vi "intersection_counter.vi"(8 "Booleanos e Contadores Iniciais":T1={"Correct"=FALSE, "Enable State change"=TRUE, "First End"=FALSE, "Intersections crossed"=0.0, "Intersections crossed total"=0.0, "Bonecos"=0.0} caption="Booleanos e Contadores") -> (2 "Intersections crossed":dbl)   [LabVIEW 2016]
uses:
  booleanos.ctl
panel:
  # "Permite que ocorra troca \nde estados se True e interrompe-as \nse False."
  # "Booleano que retorna F quando chega em Delivery.\nGarantindo que não contará\nmais intersections"
  # "Salva o total de interseções \ncruzadas"
  # "Contador de quantas \ninterseções foram cruzadas.\nSoma ao acertar"
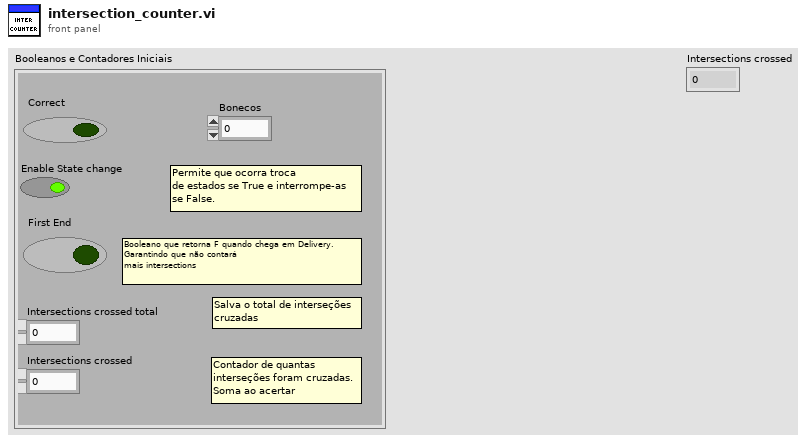
[diagram p1: front panel]
types:
  T1 = typedef "booleanos.ctl" = cluster{"Correct":bool, "Enable State change":bool, "First End":bool, "Intersections crossed":dbl, "Intersections crossed total":dbl, "Bonecos":dbl}
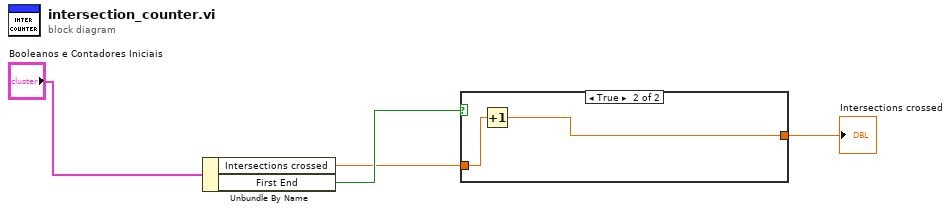
[diagram p0: block diagram]
diagram:
  n1 = Unbundle By Name("Booleanos e Contadores Iniciais") -> ("Intersections crossed"=w3:dbl, "First End"=w4:bool)
  n2 = case shown="True" w4 {
    tunnel: w3 -> [w5 w7]
    tunnel: [w5 w6] -> w2
    frame False {
    }
    frame True {
      n3 = Increment(x=w7) -> (x+1=w6:dbl)
    }
  }
  "Intersections crossed" <- w2
